vi "flare-ucoc-TEST.vi"() -> ()   [LabVIEW 2017]
uses:
  mqtt-LabVIEW/src/class/mqtt/mqttConfigFunction.ctl
  mqtt-LabVIEW/src/class/mqtt/mqtt.lvclass/mqtt.ctl
  mqtt-LabVIEW/src/class/mqtt/mqttTypedef/mqttSubscribeCluster.ctl
  mqtt-LabVIEW/src/class/mqtt/mqttTypedef/mqttQOSlevel.ctl
  flare_undulator/mqtt payload to double.vi
  flare_undulator/mqtt payload to boolean.vi
  mqtt-LabVIEW/src/class/mqtt/mqtt.lvclass
panel:
  in  "override killswitch":bool
  in  "brake control":bool
  out "brake":bool
  out "actual taper (mm)":dbl format="%0.3f"
  out "actual wavenumbers":dbl=100.0 format="%0.3f"
  out "actual wavelength (µm)":dbl=100.0 format="%0.3f"
  out "actual gap (mm)":dbl=24.8 min=24.6 max=310.0 format="%0.3f"
  in  "wavenumbers":dbl=100.0 format="%0.3f"
  in  "halt":bool
  in  "wavelength (µm)":dbl=100.0 min=57.09371410460931 max=842.9323988101984 format="%0.3f"
  in  "dipole current (A)":dbl=90.0
  in  "enable client time sending":bool
  in  "keep connected":bool
  in  "acceleration (mm/s²)":dbl=1.0 format="%.;%0.3f"
  in  "velocity (mm/s)":dbl=1.0 format="%.;%0.3f"
  out "down rev":bool
  out "down fwd":bool
  out "up rev":bool
  out "up fwd":bool
  in  "decelerate":bool
  in  "taper (mm)":dbl min=-5.0 max=5.0 format="%.;%0.3f"
  out "upstream gap encoder":dbl format="%.;%.3f"
  out "moving":bool
  out "state":string
  out "downstream gap encoder":dbl format="%.;%.3f"
  in  "gap (mm)":dbl=30.0 min=24.8 max=300.0 format="%0.3f"
  out "upstream motor gap":dbl format="%.; %0.3f"
  out "downstream motor gap":dbl format="%.; %0.3f"
  out "MQTT Subscribed":bool
  out "MQTT Connection":bool
  out "RX Topic":string
  out "RX Value":string
  out "messageID":u16
  out "quit":bool
  # "²%"
  # "¼%"
  # "²%"
  # "¼%"
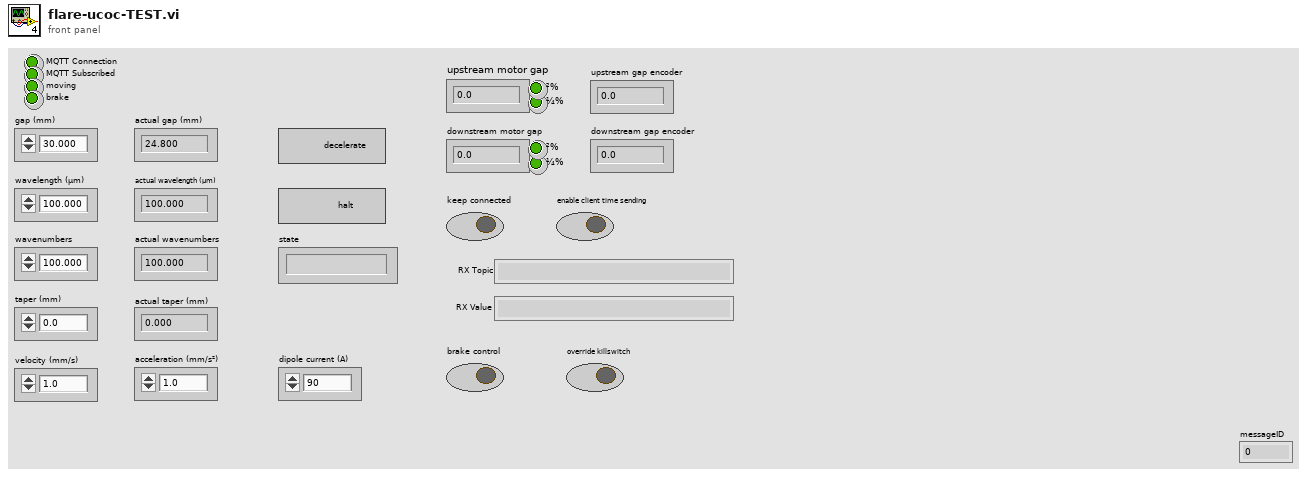
[diagram p1: front panel]
types:
  T1 = enum8{"Enabled", "Disabled", "Disabled and Grayed Out"}
  T2 = typedef "mqtt.lvclass/mqttConfigFunction.ctl" = enum16{"init", "deinit", "set", "get"}
  T3 = typedef "mqttSubscribeCluster.ctl" = cluster{"Topic":string, "QoS":T4}
  T4 = typedef "mqttQOSlevel.ctl" = enum8{"At most once", "At least once", "Exactly once", "Reserved"}
  T5 = typedef "mqttUserInformation.ctl" = cluster{"Will message":string, "Will Topic":string}
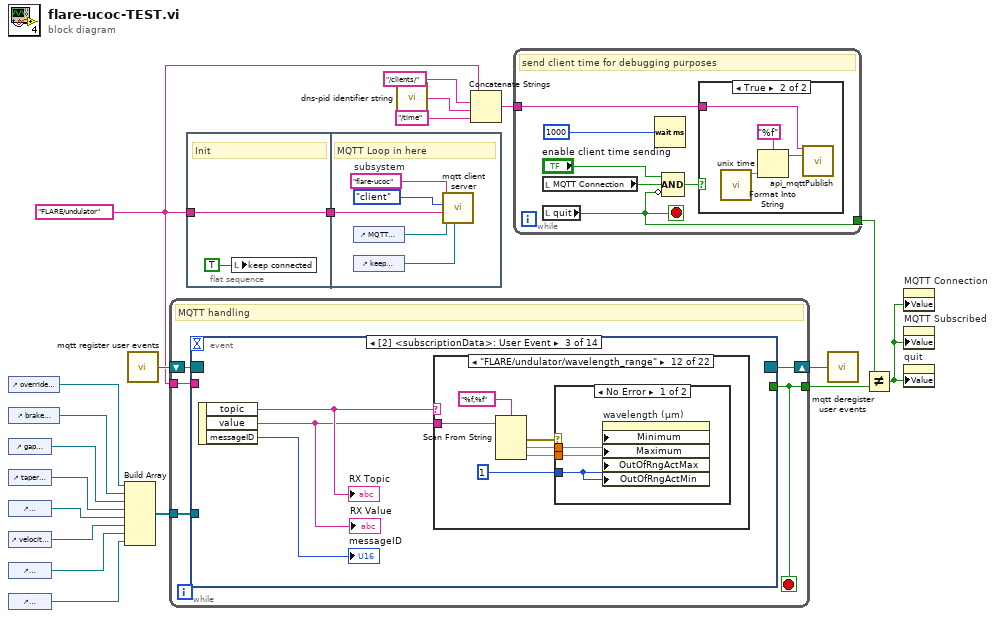
[diagram p0: block diagram]
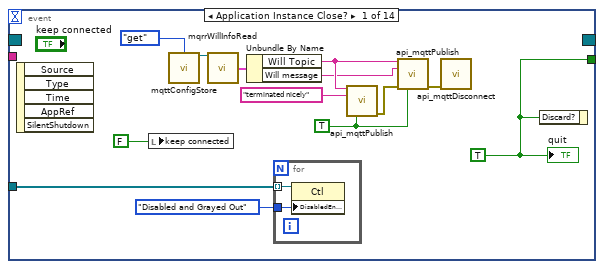
[diagram p3: hidden frame]
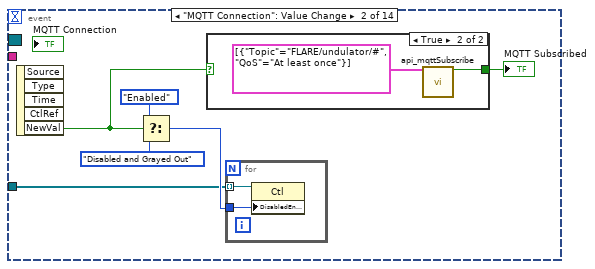
[diagram p4: hidden frame]
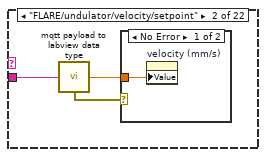
[diagram p7: hidden frame]
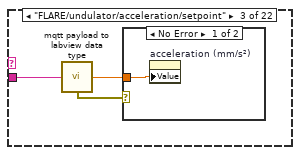
[diagram p9: hidden frame]
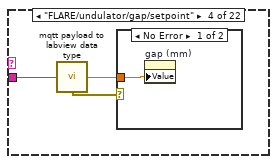
[diagram p11: hidden frame]
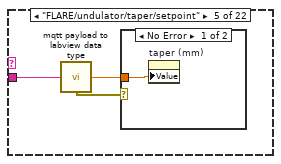
[diagram p13: hidden frame]
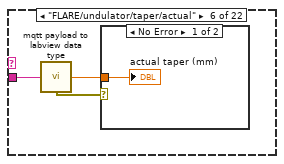
[diagram p15: hidden frame]
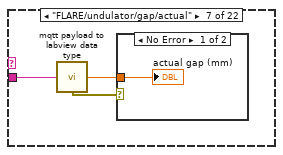
[diagram p17: hidden frame]
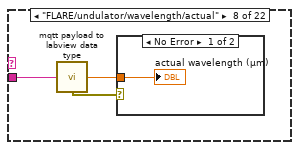
[diagram p19: hidden frame]
diagram:
  w1 = "FLARE/undulator" ("mqtt prefix")
  n1 = control-ref of="override killswitch"() -> (w3:refnum<vi>)
  n2 = control-ref of="brake control"() -> (w4:refnum<vi>)
  n3 = control-ref of="gap (mm)"() -> (w11:refnum<vi>)
  n4 = control-ref of="taper (mm)"() -> (w10:refnum<vi>)
  n5 = control-ref of="wavelength (µm)"() -> (w8:refnum<vi>)
  n6 = control-ref of="velocity (mm/s)"() -> (w7:refnum<vi>)
  n7 = control-ref of="wavenumbers"() -> (w6:refnum<vi>)
  n8 = control-ref of="acceleration (mm/s²)"() -> (w5:refnum<vi>)
  n9 = Build Array(w3, w4, w11, w10, w8, w7, w6, w5) -> (w9:refnum<vi>[])
  n10 = call "mqtt register user events.vi"() -> ("Event Registration Refnum"=w20:refnum<event-registration>)  [unwired: 1 in]
  n11 = while {
    shift-right: [w24] -> w19
    shift-left: w20 -> [w25]
    tunnel: [w23] -> w18
    tunnel: w9 -> [w22]
    tunnel: w1 -> [w21]
    stop <- w23 stop-if-true
    # "MQTT handling"
    n12 = event shown="[2] <subscriptionData>: User Event" {
      selector: w25 -> [_ _ _ _ _ _ _ _ _ _ _ _ _ _]
      dyn-events: [_ _ _ _ _ _ _ _ _ _ _ _ _ _] -> w24
      timeout: _ -> [_ _ _ _ _ _ _ _ _ _ _ _ _ _]
      tunnel: [w26 _ _ _ _ _ _ _ _ _ _ _ _ _] -> w23
      tunnel: w21 -> [_ _ _ w129 w136 w143 w151 w162 w169 w176 w183 w185 w191 w202]
      tunnel: w22 -> [w29 w43 _ _ _ _ _ _ _ _ _ _ _ _]
      event Application Instance Close? {
        w26 = TRUE ("quit")
        w30 = TRUE ("retain(F)")
        n13 = event-data() -> ()  [unwired: 1 in, 5 out]
        n14 = local write "keep connected"(FALSE ("keep connected")) -> ()
        n15 = call "mqttConfigStore.vi"("function"=mqttConfigFunction."get") -> ("mqtt.lvclass out"=w36:refnum<class "mqtt.lvclass">)  [unwired: 13 in, 1 out]
        n16 = call "mqrrWillInfoRead.vi"("mqtt in"=w36) -> ("Will Info"=w38:T5)  [unwired: 12 in, 2 out]
        n17 = Unbundle By Name(w38) -> ("Will Topic"=w32:string, "Will message"=w31:string)
        n18 = for {
          tunnel: w29 -> [w40] mode=indexing
          tunnel: T1."Disabled and Grayed Out" ("Disabled") -> [w39]
          n19 = property class="Ctl"(reference=w40, "DisabledEnum"=w39) -> ()  [unwired: 1 in, 2 out]
        }
        n20 = call "api_mqttPublish.vi"("topic"=w32, "value"="terminated nicely", "retain(F)"=w30) -> ("error out"=w34:errorcluster)  [unwired: 11 in, 1 out]
        n21 = call "api_mqttPublish.vi"("topic"=w32, "value"=w31, "error in (no error)"=w34, "retain(F)"=w30) -> ("error out"=w33:errorcluster)  [unwired: 10 in, 1 out]
        n22 = call "api_mqttDisconnect.vi"("error in (no error)"=w33) -> ()  [unwired: 13 in, 2 out]
        n23 = event-data("Discard?"=w26) -> ()  [unwired: 1 in, 1 out]
        "quit" <- w26
      }
      event "MQTT Connection": Value Change {
        n24 = event-data() -> ("NewVal"=w42:bool)  [unwired: 1 in, 4 out]
        n25 = Select(t=T1."Enabled" ("Disabled"), s=w42, f=T1."Disabled and Grayed Out") -> (s? t:f=w44:T1)
        n26 = case shown="True" w42 {
          selector: w42 -> [w47 _]
          tunnel: [w47 w48] -> w41
          frame False {
          }
          frame True {
            n27 = call "api_mqttSubscribe.vi"("subscriptionInfo"=T3[] [{"Topic"="FLARE/undulator/#", "QoS"=enum."At least once"}] ("subscriptionInfo 2")) -> ("success"=w48:bool)  [unwired: 13 in, 1 out]
          }
        }
        "MQTT Subscribed" <- w41
        n28 = for {
          tunnel: w43 -> [w51] mode=indexing
          tunnel: w44 -> [w50]
          n29 = property class="Ctl"(reference=w51, "DisabledEnum"=w50) -> ()  [unwired: 1 in, 2 out]
        }
      }
      event User Event {
        n30 = event-data() -> ("topic"=w53:string, "value"=w52:string, "messageID"=→"messageID":u16)  [unwired: 1 in]
        "RX Topic" <- w53
        "RX Value" <- w52
        n31 = case shown="\"FLARE/undulator/wavelength_range\"" w53 {
          tunnel: w52 -> [_ w57 w61 w65 w69 w73 w77 w81 w85 w89 w91 w100 w105 w106 w108 w111 w114 w118 w122 w124 w126 w128]
          frame "False", Default {
          }
          frame "FLARE/undulator/velocity/setpoint" {
            n32 = call-poly "mqtt payload to labview data type.vi"("MQTT payload"=w57) -> ("double"=w56:dbl, "error out"=w55:errorcluster)  [unwired: 13 in]
            n33 = case shown="No Error" w55 {
              tunnel: w56 -> [w58 _]
              frame No Error {
                n34 = property on="velocity (mm/s)" class="DigNum (strict)"("Value"=w58) -> ()  [unwired: 2 in, 2 out]
              }
              frame Error {
              }
            }
          }
          frame "FLARE/undulator/acceleration/setpoint" {
            n35 = call-poly "mqtt payload to labview data type.vi"("MQTT payload"=w61) -> ("double"=w60:dbl, "error out"=w59:errorcluster)  [unwired: 13 in]
            n36 = case shown="No Error" w59 {
              tunnel: w60 -> [w62 _]
              frame No Error {
                n37 = property on="acceleration (mm/s²)" class="DigNum (strict)"("Value"=w62) -> ()  [unwired: 2 in, 2 out]
              }
              frame Error {
              }
            }
          }
          frame "FLARE/undulator/gap/setpoint" {
            n38 = call-poly "mqtt payload to labview data type.vi"("MQTT payload"=w65) -> ("double"=w64:dbl, "error out"=w63:errorcluster)  [unwired: 13 in]
            n39 = case shown="No Error" w63 {
              tunnel: w64 -> [w66 _]
              frame No Error {
                n40 = property on="gap (mm)" class="DigNum (strict)"("Value"=w66) -> ()  [unwired: 2 in, 2 out]
              }
              frame Error {
              }
            }
          }
          frame "FLARE/undulator/taper/setpoint" {
            n41 = call-poly "mqtt payload to labview data type.vi"("MQTT payload"=w69) -> ("double"=w68:dbl, "error out"=w67:errorcluster)  [unwired: 13 in]
            n42 = case shown="No Error" w67 {
              tunnel: w68 -> [w70 _]
              frame No Error {
                n43 = property on="taper (mm)" class="DigNum (strict)"("Value"=w70) -> ()  [unwired: 2 in, 2 out]
              }
              frame Error {
              }
            }
          }
          frame "FLARE/undulator/taper/actual" {
            n44 = call-poly "mqtt payload to labview data type.vi"("MQTT payload"=w73) -> ("double"=w72:dbl, "error out"=w71:errorcluster)  [unwired: 13 in]
            n45 = case shown="No Error" w71 {
              tunnel: w72 -> [w74 _]
              frame No Error {
                "actual taper (mm)" <- w74
              }
              frame Error {
              }
            }
          }
          frame "FLARE/undulator/gap/actual" {
            n46 = call-poly "mqtt payload to labview data type.vi"("MQTT payload"=w77) -> ("double"=w76:dbl, "error out"=w75:errorcluster)  [unwired: 13 in]
            n47 = case shown="No Error" w75 {
              tunnel: w76 -> [w78 _]
              frame No Error {
                "actual gap (mm)" <- w78
              }
              frame Error {
              }
            }
          }
          frame "FLARE/undulator/wavelength/actual" {
            n48 = call-poly "mqtt payload to labview data type.vi"("MQTT payload"=w81) -> ("double"=w80:dbl, "error out"=w79:errorcluster)  [unwired: 13 in]
            n49 = case shown="No Error" w79 {
              tunnel: w80 -> [w82 _]
              frame No Error {
                "actual wavelength (µm)" <- w82
              }
              frame Error {
              }
            }
          }
          frame "FLARE/undulator/wavenumbers/actual" {
            n50 = call-poly "mqtt payload to labview data type.vi"("MQTT payload"=w85) -> ("double"=w84:dbl, "error out"=w83:errorcluster)  [unwired: 13 in]
            n51 = case shown="No Error" w83 {
              tunnel: w84 -> [w86 _]
              frame No Error {
                "actual wavenumbers" <- w86
              }
              frame Error {
              }
            }
          }
          frame "FLARE/undulator/dipole_current" {
            n52 = call-poly "mqtt payload to labview data type.vi"("MQTT payload"=w89) -> ("double"=w88:dbl, "error out"=w87:errorcluster)  [unwired: 13 in]
            n53 = case shown="No Error" w87 {
              tunnel: w88 -> [w90 _]
              frame No Error {
                n54 = property on="dipole current (A)" class="DigNum (strict)"("Value"=w90) -> ()  [unwired: 2 in, 2 out]
              }
              frame Error {
              }
            }
          }
          frame "FLARE/undulator/downstream/gap" {
            n55 = call-poly "mqtt payload to labview data type.vi"("MQTT payload"=w91) -> ("double"=w93:dbl, "error out"=w92:errorcluster)  [unwired: 13 in]
            n56 = case shown="No Error" w92 {
              tunnel: w93 -> [w94 _]
              frame No Error {
                "downstream motor gap" <- w94
              }
              frame Error {
              }
            }
          }
          frame "FLARE/undulator/wavelength_range" {
            n57 = Scan From String(format string="%f,%f", input string=w100) -> (error out=w95:errorcluster, output 1=w98:dbl, output 2=w97:dbl)  [unwired: 4 in, 2 out]
            n58 = case shown="No Error" w95 {
              tunnel: w98 -> [w103 _]
              tunnel: w97 -> [w102 _]
              tunnel: u8 1 ("Response to Value Outside Limits:Maximum") -> [w101 _]
              frame No Error {
                n59 = property on="wavelength (µm)" class="DigNum (strict)"("Minimum"=w103, "Maximum"=w102, "OutOfRngActMax"=w101, "OutOfRngActMin"=w101) -> ()  [unwired: 2 in, 2 out]
              }
              frame Error {
              }
            }
          }
          frame "FLARE/undulator/upstream/forward_limit_active" {
            n60 = call-poly "mqtt payload to labview data type.vi"("String"=w105) -> ("Boolean"=→"up fwd":bool)  [unwired: 13 in, 1 out]
          }
          frame "FLARE/undulator/upstream/reverse_limit_active" {
            n61 = call-poly "mqtt payload to labview data type.vi"("String"=w106) -> ("Boolean"=→"up rev":bool)  [unwired: 13 in, 1 out]
          }
          frame "FLARE/undulator/downstream/forward_limit_active" {
            n62 = call-poly "mqtt payload to labview data type.vi"("String"=w108) -> ("Boolean"=→"down fwd":bool)  [unwired: 13 in, 1 out]
          }
          frame "FLARE/undulator/downstream/reverse_limit_active" {
            n63 = call-poly "mqtt payload to labview data type.vi"("String"=w111) -> ("Boolean"=→"down rev":bool)  [unwired: 13 in, 1 out]
          }
          frame "FLARE/undulator/upstream/gap" {
            n64 = call-poly "mqtt payload to labview data type.vi"("MQTT payload"=w114) -> ("double"=w113:dbl, "error out"=w112:errorcluster)  [unwired: 13 in]
            n65 = case shown="No Error" w112 {
              tunnel: w113 -> [w115 _]
              frame No Error {
                "upstream motor gap" <- w115
              }
              frame Error {
              }
            }
          }
          frame "FLARE/undulator/downstream/encoder/gap" {
            n66 = call-poly "mqtt payload to labview data type.vi"("MQTT payload"=w118) -> ("double"=w117:dbl, "error out"=w116:errorcluster)  [unwired: 13 in]
            n67 = case shown="No Error" w116 {
              tunnel: w117 -> [w119 _]
              frame No Error {
                "downstream gap encoder" <- w119
              }
              frame Error {
              }
            }
          }
          frame "FLARE/undulator/upstream/encoder/gap" {
            n68 = call-poly "mqtt payload to labview data type.vi"("MQTT payload"=w122) -> ("double"=w121:dbl, "error out"=w120:errorcluster)  [unwired: 13 in]
            n69 = case shown="No Error" w120 {
              tunnel: w121 -> [w123 _]
              frame No Error {
                "upstream gap encoder" <- w123
              }
              frame Error {
              }
            }
          }
          frame "FLARE/undulator/state" {
            "state" <- w124
          }
          frame "FLARE/undulator/moving" {
            n70 = call-poly "mqtt payload to labview data type.vi"("String"=w126) -> ("Boolean"=→"moving":bool)  [unwired: 13 in, 1 out]
          }
          frame "FLARE/undulator/brake" {
            n71 = call-poly "mqtt payload to labview data type.vi"("String"=w128) -> ("Boolean"=w127:bool)  [unwired: 13 in, 1 out]
            "brake" <- w127
            n72 = property on="brake control" class="Bool (strict)"("Value"=w127) -> ()  [unwired: 2 in, 2 out]
          }
        }
      }
      event "brake control": Value Change {
        n73 = event-data() -> ("NewVal"=w133:bool)  [unwired: 1 in, 5 out]
        n74 = Select(t="True" ("string"), s=w133, f="False" ("string")) -> (s? t:f=w130:string)
        n75 = Concatenate Strings(w129, "/brake/cmd" ("string")) -> (w135:string)
        n76 = call "api_mqttPublish.vi"("topic"=w135, "value"=w130) -> ()  [unwired: 12 in, 2 out]
      }
      event "override killswitch": Value Change {
        n77 = event-data() -> ("NewVal"=w140:bool)  [unwired: 1 in, 5 out]
        n78 = Select(t="True" ("string"), s=w140, f="False" ("string")) -> (s? t:f=w137:string)
        n79 = Concatenate Strings(w136, "/killswitch_override/cmd" ("string")) -> (w142:string)
        n80 = call "api_mqttPublish.vi"("topic"=w142, "value"=w137) -> ()  [unwired: 12 in, 2 out]
      }
      event "wavelength (µm)": Value Change {
        n81 = event-data() -> ()  [unwired: 1 in, 6 out]
        n82 = Concatenate Strings(w143, "/wavelength/setpoint" ("string")) -> (w148:string)
        n83 = Format Into String(format string="%.;%f", "wavelength (µm)") -> (resulting string=w147:string)  [unwired: 2 in, 1 out]
        n84 = call "api_mqttPublish.vi"("topic"=w148, "value"=w147) -> ()  [unwired: 12 in, 2 out]
      }
      event "dipole current (A)": Value Change {
        n85 = event-data() -> ()  [unwired: 1 in, 6 out]
        n86 = Format Into String(format string="%.;%f", "dipole current (A)") -> (resulting string=w154:string)  [unwired: 2 in, 1 out]
        n87 = Concatenate Strings(w151, "/dipole_current" ("string")) -> (w155:string)
        n88 = call "api_mqttPublish.vi"("topic"=w155, "value"=w154, "retain(F)"=TRUE) -> ()  [unwired: 11 in, 2 out]
      }
      event "gap (mm)": Value Change {
        n89 = event-data() -> ()  [unwired: 1 in, 6 out]
        n90 = Format Into String(format string="%.;%f", "gap (mm)") -> (resulting string=w159:string)  [unwired: 2 in, 1 out]
        n91 = Concatenate Strings(w162, "/gap/setpoint" ("string")) -> (w161:string)
        n92 = call "api_mqttPublish.vi"("topic"=w161, "value"=w159, "retain(F)"=TRUE) -> ()  [unwired: 11 in, 2 out]
      }
      event "wavenumbers": Value Change {
        n93 = event-data() -> ()  [unwired: 1 in, 6 out]
        n94 = Format Into String(format string="%.;%f", "wavenumbers") -> (resulting string=w167:string)  [unwired: 2 in, 1 out]
        n95 = Concatenate Strings(w169, "/wavenumbers/setpoint" ("string")) -> (w168:string)
        n96 = call "api_mqttPublish.vi"("topic"=w168, "value"=w167, "retain(F)"=TRUE) -> ()  [unwired: 11 in, 2 out]
      }
      event "acceleration (mm/s²)": Value Change {
        n97 = event-data() -> ()  [unwired: 1 in, 6 out]
        n98 = Format Into String(format string="%.;%f", "acceleration (mm/s²)") -> (resulting string=w174:string)  [unwired: 2 in, 1 out]
        n99 = Concatenate Strings(w176, "/acceleration/setpoint" ("string")) -> (w175:string)
        n100 = call "api_mqttPublish.vi"("topic"=w175, "value"=w174, "retain(F)"=TRUE) -> ()  [unwired: 11 in, 2 out]
      }
      event "velocity (mm/s)": Value Change {
        n101 = event-data() -> ()  [unwired: 1 in, 6 out]
        n102 = Format Into String(format string="%.;%f", "velocity (mm/s)") -> (resulting string=w181:string)  [unwired: 2 in, 1 out]
        n103 = Concatenate Strings(w183, "/velocity/setpoint" ("string")) -> (w182:string)
        n104 = call "api_mqttPublish.vi"("topic"=w182, "value"=w181, "retain(F)"=TRUE) -> ()  [unwired: 11 in, 2 out]
      }
      event "decelerate": Value Change {
        n105 = event-data() -> ("NewVal"=w184:bool)  [unwired: 1 in, 5 out]
        n106 = case shown="True" w184 {
          tunnel: w185 -> [_ w189]
          frame False {
          }
          frame True {
            n107 = Concatenate Strings(w189, "/stop" ("string")) -> (w188:string)
            n108 = call "api_mqttPublish.vi"("topic"=w188, "value"="decelerate" ("string")) -> ()  [unwired: 12 in, 2 out]
          }
        }
      }
      event "halt": Value Change {
        n109 = event-data() -> ("NewVal"=w190:bool)  [unwired: 1 in, 5 out]
        n110 = case shown="True" w190 {
          tunnel: w191 -> [_ w195]
          frame False {
          }
          frame True {
            n111 = Concatenate Strings(w195, "/stop" ("string")) -> (w194:string)
            n112 = call "api_mqttPublish.vi"("topic"=w194, "value"="halt" ("string")) -> ()  [unwired: 12 in, 2 out]
          }
        }
      }
      event "taper (mm)": Value Change {
        n113 = event-data() -> ()  [unwired: 1 in, 6 out]
        n114 = Format Into String(format string="%.;%f", "taper (mm)") -> (resulting string=w200:string)  [unwired: 2 in, 1 out]
        n115 = Concatenate Strings(w202, "/taper/setpoint" ("string")) -> (w201:string)
        n116 = call "api_mqttPublish.vi"("topic"=w201, "value"=w200, "retain(F)"=TRUE) -> ()  [unwired: 11 in, 2 out]
      }
    }
  }
  n117 = flat-sequence {
    tunnel: [w203] -> w2
    tunnel: w1 -> [w203]
    tunnel: w2 -> [w207]
    frame #0 {
      # "Init"
      n118 = local write "keep connected"(TRUE ("keep connected")) -> ()
    }
    frame #1 {
      w205 = "flare-ucoc"  # subsystem
      # "MQTT Loop in here"
      n119 = control-ref of="MQTT Connection"() -> (w208:refnum<vi>)
      n120 = control-ref of="keep connected"() -> (w209:refnum<vi>)
      n121 = call "mqtt client server.vi"("keep connected"=w209, "connect success reference"=w208, "mqtt prefix"=w207, "client or server"=enum16{"client", "server"}."client", "subsystem"=w205) -> ()  [unwired: 6 in, 1 out]
    }
  }
  n122 = call "dns-pid identifier string.vi"() -> ("DNS_PID Identifier string"=w15:string)  [unwired: 1 in]
  n123 = Concatenate Strings(w1, "/clients/" ("string"), w15, "/time" ("string")) -> (w13:string)
  n124 = while {
    tunnel: [w211] -> w17
    tunnel: w13 -> [w212]
    stop <- w211 stop-if-true
    # "send client time for debugging purposes"
    n125 = local read "MQTT Connection"() -> (w214:bool)
    n126 = local read "quit"() -> (w211:bool)
    n127 = Wait (ms)(milliseconds to wait=u32 1000) -> ()  [unwired: 1 out]
    n128 = Compound Arithmetic op=AND("enable client time sending", w214, invert w211) -> (w213:bool)
    n129 = case shown="True" w213 {
      tunnel: w212 -> [_ w216]
      frame False {
      }
      frame True {
        n130 = call "unix time.vi"() -> ("Unix time"=w218:dbl)  [unwired: 10 in, 1 out]
        n131 = Format Into String(format string="%f", w218) -> (resulting string=w217:string)  [unwired: 2 in, 1 out]
        n132 = call "api_mqttPublish.vi"("topic"=w216, "value"=w217) -> ()  [unwired: 12 in, 2 out]
      }
    }
  }
  n133 = call "mqtt deregister user events.vi"("Event Registration Refnum in"=w19) -> ()  [unwired: 1 in]
  n134 = Not Equal?(x=w17, y=w18) -> (x != y?=w12:bool)
  n135 = property on="MQTT Connection" class="Bool (strict)"("Value"=w12) -> ()  [unwired: 2 in, 2 out]
  n136 = property on="MQTT Subscribed" class="Bool (strict)"("Value"=w12) -> ()  [unwired: 2 in, 2 out]
  n137 = property on="quit" class="Bool (strict)"("Value"=w12) -> ()  [unwired: 2 in, 2 out]
